vi "Get Logout Path.vi"(8 "error in (no error)":errorcluster, 11 "FormAuthentication in":refnum<class "FormAuthentication.lvclass">) -> (0 "error out":errorcluster, 2 "Logout Path":string, 3 "FormAuthentication out":refnum<class "FormAuthentication.lvclass">)   [LabVIEW 2020, in "HTTP Server.lvlib" / "FormAuthentication.lvclass"]
uses:
  FormAuthentication.lvclass
  FormAuthentication.lvclass/FormAuthentication.ctl
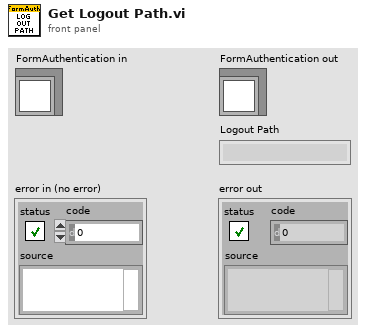
[diagram p1: front panel]
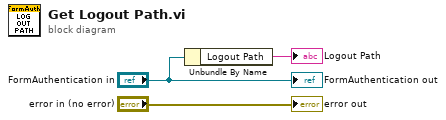
[diagram p0: block diagram]
diagram:
  n1 = Unbundle By Name("FormAuthentication in") -> ("Logout Path"=→"Logout Path":string)
  "error out" <- "error in (no error)"
  "FormAuthentication out" <- "FormAuthentication in"
